vi "Obtain and Register Queue.vi"(7 "max queue size (-1, unlimited)":i32=-1, 8 "error in (no error)":errorcluster, 9 "create if not found? (T)":bool=TRUE, 11 "Queue Name (unnamed)":string) -> (0 "error out":errorcluster, 3 "Queue Reference":refnum<queue>)   [LabVIEW 2021]
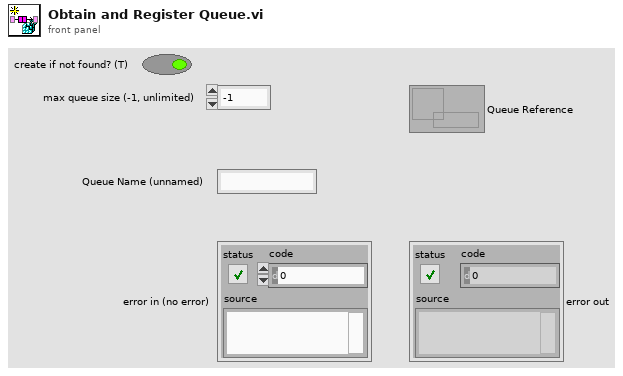
[diagram p1: front panel]
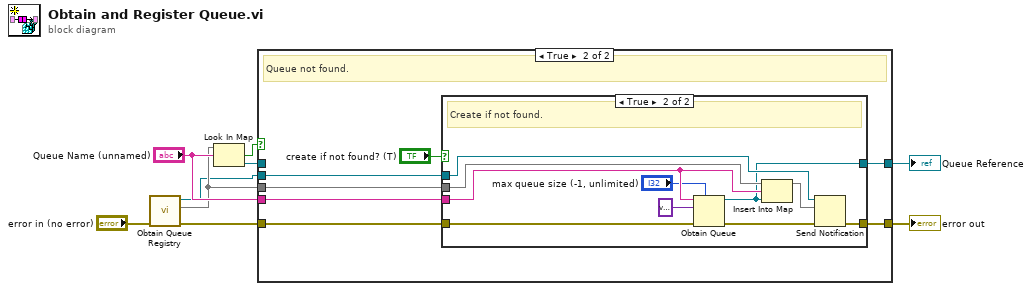
[diagram p0: block diagram]
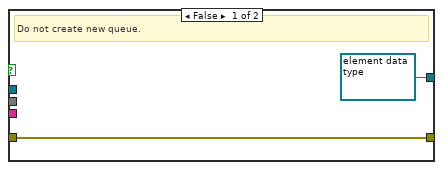
[diagram p3: hidden frame]
diagram:
  n1 = call "Obtain Queue Registry.vi"("error in (no error)"="error in (no error)") -> ("error out"=w3:errorcluster, "Queue Registry"=w2:map{string, refnum<queue>}, "Queue Registry Notifier"=w1:refnum<notifier>)  [unwired: 8 in]
  n2 = Look In Map(map=w2, key="Queue Name (unnamed)") -> (key not found?=w4:bool, value=w6:refnum<queue>)  [unwired: 1 in]
  n3 = case shown="True" w4 {
    tunnel: "Queue Name (unnamed)" -> [_ w16]
    tunnel: w3 -> [w10 w18]
    tunnel: w2 -> [_ w17]
    tunnel: w6 -> [w11 _]
    tunnel: [w11 w14] -> w7
    tunnel: w1 -> [_ w15]
    tunnel: [w10 w13] -> w9
    frame False {
      # "Queue found."
    }
    frame True {
      # "Queue not found."
      n4 = case shown="True" "create if not found? (T)" {
        tunnel: w18 -> [w19 w29]
        tunnel: w17 -> [_ w28]
        tunnel: w16 -> [_ w27]
        tunnel: w15 -> [_ w26]
        tunnel: [refnum<queue> refnum ("queue out") w23] -> w14
        tunnel: [w19 w22] -> w13
        frame False {
          # "Do not create new queue."
        }
        frame True {
          # "Create if not found."
          n5 = Obtain Queue(max queue size (-1, unlimited)="max queue size (-1, unlimited)", name (unnamed)=w27, element data type=variant, error in (no error)=w29) -> (queue out=w23:refnum<queue>, error out=w24:errorcluster)  [unwired: 1 in, 1 out]
          n6 = Insert Into Map(map in=w28, key=w27, value=w23) -> (map out=w25:map{string, refnum<queue>})  [unwired: 2 out]
          n7 = Send Notification(notification=w25, notifier=w26, error in (no error)=w24) -> (error out=w22:errorcluster)  [unwired: 1 out]
        }
      }
    }
  }
  "Queue Reference" <- w7
  "error out" <- w9
